vi "Mouse Down.vi"(7 "Map Model in":refnum<class "Map Model.lvclass">, 8 "error in (no error)":errorcluster, 10 "Position":T1, 11 "Eraser in":refnum<class "Eraser.lvclass">) -> (0 "error out":errorcluster, 3 "Eraser out":refnum<class "Eraser.lvclass">, 5 "Map Model out":refnum<class "Map Model.lvclass">)   [LabVIEW 2020, in "Map Model.lvlib" / "Eraser.lvclass"]
uses:
  Eraser.lvclass
  <vilib>/Utility/miscctls.llb/LVPoint32TypeDef.ctl
  Map Model/Map Model.lvclass
  Map Model/Map Model.lvclass/Map Model.ctl
  Undoable Tool/Undoable Tool.lvclass
panel:
  # "NOTICE -- YOU MUST LEAVE THIS NOTICE IN PLACE.\n\nCopyright (c) 2017, LIANG LIU Shawn.Liu.cn@gmail.com\nAll rights reserved.\n\nRedistribution and use in source and binary forms, with or without modification, are permitted provided that the following conditions are met:\n-Redistributions of source code must retain the above copyright notice, this list of conditions and the following disclaimer.\n-Redistributions in binary form must reproduce the above copyright notice, this list of conditions and the following disclaimer in the documentation and/or other materials provided with the distribution.\n-Neither the name of the eLp nor the names of its contributors may be used to endorse or promote products derived from this software without specific prior written permission.\n\nTHIS SOFTWARE IS PROVIDED BY THE COPYRIGHT HOLDERS AND CONTRIBUTORS \"AS IS\" AND ANY EXPRESS OR IMPLIED WARRANTIES, INCLUDING, BUT NOT LIMITED TO, THE IMPLIED WARRANTIES OF MERCHANTABILITY AND FITNESS FOR A PARTICULAR PURPOSE ARE DISCLAIMED. IN NO EVENT SHALL THE COPYRIGHT HOLDER OR CONTRIBUTORS BE LIABLE FOR ANY DIRECT, INDIRECT, INCIDENTAL, SPECIAL, EXEMPLARY, OR CONSEQUENTIAL DAMAGES (INCLUDING, BUT NOT LIMITED TO, PROCUREMENT OF SUBSTITUTE GOODS OR SERVICES; LOSS OF USE, DATA, OR PROFITS; OR BUSINESS INTERRUPTION) HOWEVER CAUSED AND ON ANY THEORY OF LIABILITY, WHETHER IN CONTRACT, STRICT LIABILITY, OR TORT (INCLUDING NEGLIGENCE OR OTHERWISE) ARISING IN ANY WAY OUT OF THE USE OF THIS SOFTWARE, EVEN IF ADVISED OF THE POSSIBILITY OF SUCH DAMAGE."
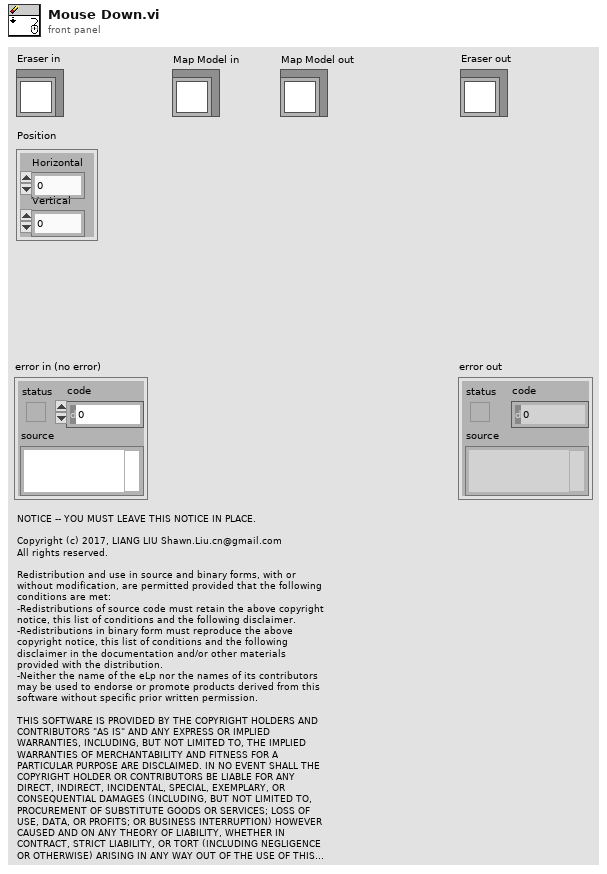
[diagram p1: front panel]
types:
  T1 = typedef "LVPoint32TypeDef.ctl" = cluster{"Horizontal":i32, "Vertical":i32}
  T2 = cluster{"Width":u16, "Style":enum32{"Solid", "Dash", "Dot", "DashDot", "DashDotDot"}}
  T3 = cluster{"Occupied Color":cluster{"Value":u8, "Color":u32}, "Free Color":cluster{"Value":u8, "Color":u32}, "Unknown Color":cluster{"Value":u8, "Color":u32}}
  T4 = typedef "LVPointTypeDef.ctl" = cluster{"Horizontal":i16, "Vertical":i16}
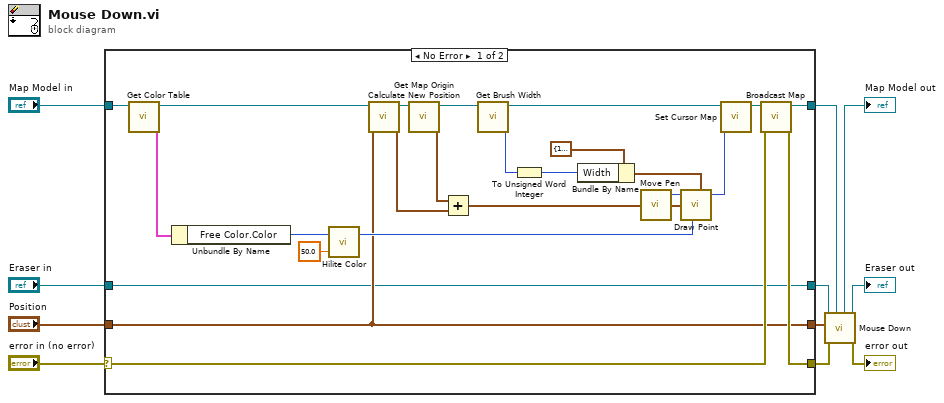
[diagram p0: block diagram]
diagram:
  n1 = case shown="No Error" "error in (no error)" {
    selector: "error in (no error)" -> [w34 w39]
    tunnel: "Map Model in" -> [w35 w38]
    tunnel: [w33 w38] -> w8
    tunnel: [w32 w39] -> w5
    tunnel: "Position" -> [w14 w36]
    tunnel: [w14 w36] -> w3
    tunnel: [w13 w37] -> w2
    tunnel: "Eraser in" -> [w13 w37]
    frame No Error {
      n2 = call "Get Color Table.vi"("Map Model in"=w35) -> ("Color Table"=w26:T3, "Map Model out"=w27:refnum<class "Map Model.lvclass">)  [unwired: 9 in]
      n3 = Unbundle By Name(w26) -> ("Free Color.Color"=w25:u32)
      n4 = call <vilib>:"Hilite Color.vi"("Percentage(30)"=50.0, "Color In"=w25) -> ("Hilite"=w19:u32)  [unwired: 1 out]
      n5 = call "Calculate New Position.vi"("Position in"=w14, "Map Model in"=w27) -> ("Position out"=w15:T1, "Map Model out"=w16:refnum<class "Map Model.lvclass">)  [unwired: 8 in]
      n6 = call "Get Map Origin.vi"("Map Model in"=w16) -> ("Map Origin"=w17:T4, "Map Model out"=w18:refnum<class "Map Model.lvclass">)  [unwired: 9 in]
      n7 = Add(x=w17, y=w15) -> (x+y=w12:T1)
      n8 = call "Get Brush Width.vi"("Map Model in"=w18) -> ("Brush Width"=w24:i32, "Map Model out"=w29:refnum<class "Map Model.lvclass">)  [unwired: 9 in]
      n9 = To Unsigned Word Integer(number=w24) -> (unsigned 16bit integer=w23:u16)
      n10 = Bundle By Name(cluster=T2 {"Width"=1, "Style"=enum."Solid"} ("pen"), "Width"=w23) -> (w20:T2)
      n11 = call <vilib>:"Move Pen.vi"("new position"=w12) -> ("new picture"=w30:picture)  [unwired: 4 in]
      n12 = call <vilib>:"Draw Point.vi"("picture"=w30, "point(x,y)"=w12, "color(black)"=w19, "pen"=w20) -> ("new picture"=w21:picture)  [unwired: 5 in]
      n13 = call "Set Cursor Map.vi"("Cursor Map"=w21, "Map Model in"=w29) -> ("Map Model out"=w31:refnum<class "Map Model.lvclass">)  [unwired: 9 in]
      n14 = call "Broadcast Map.vi"("error in (no error)"=w34, "Map Model in"=w31) -> ("error out"=w32:errorcluster, "Map Model out"=w33:refnum<class "Map Model.lvclass">)  [unwired: 8 in]
    }
    frame Error {
    }
  }
  n15 = call-parent "Mouse Down.vi"("Map Model in"=w8, "error in (no error)"=w5, "Position"=w3, "Undoable Tool in"=w2) -> ("error out"=→"error out":errorcluster, "Undoable Tool out"=→"Eraser out":refnum<class "Eraser.lvclass">, "Map Model out"=→"Map Model out":refnum<class "Map Model.lvclass">)  [unwired: 5 in]
